vi "Close Image.vi"(8 "error in (no error)":errorcluster) -> (0 "error out":errorcluster)   [LabVIEW 2018, in "Image Management.lvlib"]
uses:
  Image Management.lvlib
  Action.ctl
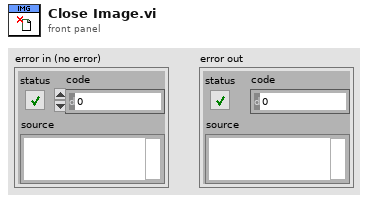
[diagram p1: front panel]
types:
  T1 = typedef "Image Management.lvlib/Action.ctl" = enum16{"Init", "Output Image Path", "Open Image in Default Program", "Find Linespaces", "Get Image Size (pixels)", "Draw ROIs", "Make Section Images", "Close"}
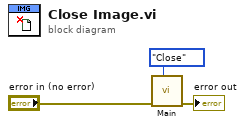
[diagram p0: block diagram]
diagram:
  n1 = call "Main.vi"("Action"=Action."Close", "Error In"="error in (no error)") -> ("Error Out"=→"error out":errorcluster)  [unwired: 8 in, 1 out]
